vi "Test Upload to S3.vi"() -> ()   [LabVIEW 2016, in "Control Experiment SM.lvclass"]
uses:
  Control Experiment SM.lvclass
panel:
  in  "file to upload":path
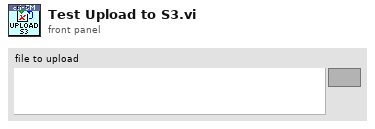
[diagram p1: front panel]
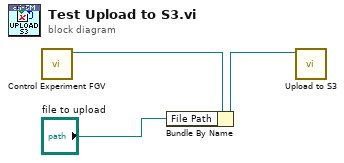
[diagram p0: block diagram]
diagram:
  n1 = call "Control Experiment FGV.vi"() -> ("Control Experiment.lvclass out"=w3:refnum<class "Control Experiment SM.lvclass">)  [unwired: 10 in, 1 out]
  n2 = Bundle By Name(cluster=w3, "File Path"="file to upload") -> (w1:refnum<class "Control Experiment SM.lvclass">)
  n3 = call "Upload to S3.vi"("Control Experiment in"=w1) -> ()  [unwired: 9 in, 2 out]
